vi "event.vi"() -> ()   [LabVIEW 2018]
panel:
  out "Repeat count":i32
  in  "Hi, print":bool
  out "String":string
  in  "stop":bool
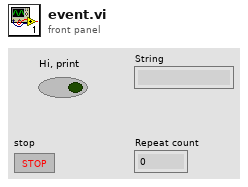
[diagram p1: front panel]
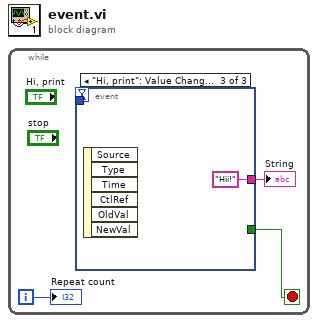
[diagram p0: block diagram]
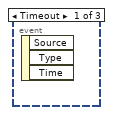
[diagram p2: hidden frame]
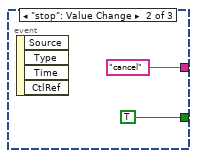
[diagram p3: hidden frame]
diagram:
  n1 = while {
    i -> [w1]
    stop <- w3 stop-if-true
    n2 = event shown="[2] \"Hi, print\": Value Change" {
      selector: _ -> [_ _ _]
      dyn-events: _ -> [_ _ _]
      timeout: _ -> [_ _ w7]
      tunnel: [_ TRUE _] -> w3
      tunnel: [_ "cancel" "Hii!"] -> w2
      tunnel: [_ _ w7] -> _
      event Timeout {
        n3 = event-data() -> ()  [unwired: 1 in, 3 out]
      }
      event "stop": Value Change {
        n4 = event-data() -> ()  [unwired: 1 in, 4 out]
      }
      event "Hi, print": Value Change {
        n5 = event-data() -> ()  [unwired: 1 in, 6 out]
      }
    }
    "String" <- w2
    "Repeat count" <- w1
  }
